vi "Test_PublishI32_PubBeforeSub_OK.vi"(8 "error in (no error)":errorcluster, 11 "TestMediator In":refnum<class "TestMediator.lvclass">) -> (0 "error out":errorcluster, 3 "TestMediator Out":refnum<class "TestMediator.lvclass">)   [LabVIEW 2015, in "TestMediator.lvclass"]
uses:
  TestMediator.lvclass
  Mediator/Mediator.lvclass
  Transport/QueueTransport/QueueTransport.lvclass/QueueTransport.ctl
  SubscriptionPolicy/BasicSubscription/BasicSubscription.lvclass/BasicSubscription.ctl
  IMediator/SubscriptionRequest/SubscriptionRequest.lvclass/SubscriptionRequest.ctl
  IMediator/IMediator Messages/Publish Msg/Publish Msg.lvclass/Publish Msg.ctl
  <vilib>/ActorFramework/Message Enqueuer/Message Enqueuer.lvclass/Message Enqueuer.ctl
  IMediator/IMediator Messages/Subscribe Msg/Subscribe Msg.lvclass/Subscribe Msg.ctl
  <vilib>/ActorFramework/Message Enqueuer/Enqueue.vi
  <vilib>/ActorFramework/Message Priority Queue/Priority Enqueue.vi
  <vilib>/Utility/error.llb/Error Cluster From Error Code.vi
  SubscriptionPolicy/BasicSubscription/BasicSubscription.lvclass
  IMediator/IMediator Messages/Publish Msg/Publish Msg.lvclass
  Transport/QueueTransport/QueueTransport.lvclass
  IMediator/SubscriptionRequest/SubscriptionRequest.lvclass
  IMediator/IMediator Messages/Subscribe Msg/Subscribe Msg.lvclass
  <vilib>/ActorFramework/Stop Msg/Stop Msg.lvclass
  <vilib>/addons/_JKI Toolkits/VI Tester/TestCase.llb/TestCase.lvclass
  <vilib>/ActorFramework/Actor/Actor.lvclass
  IMediator/ISubscriptionPolicy/ISubscriptionPolicy.lvclass
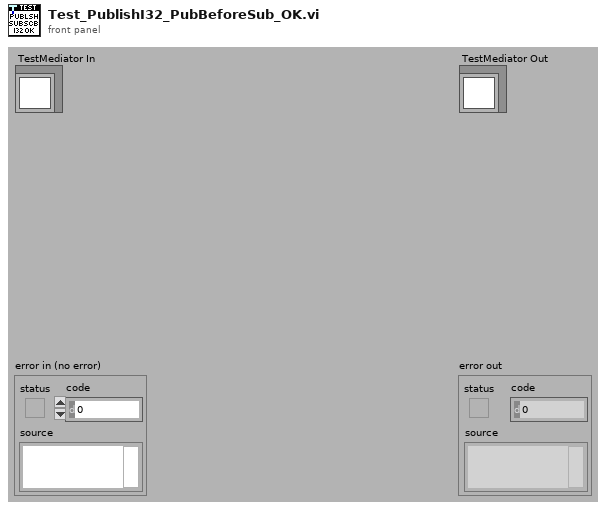
[diagram p1: front panel]
types:
  T1 = typedef "IMediator.lvlib/ISubscriptionPolicy.lvclass/ISubscriptionPolicy Reference.ctl" = refnum<data-value>
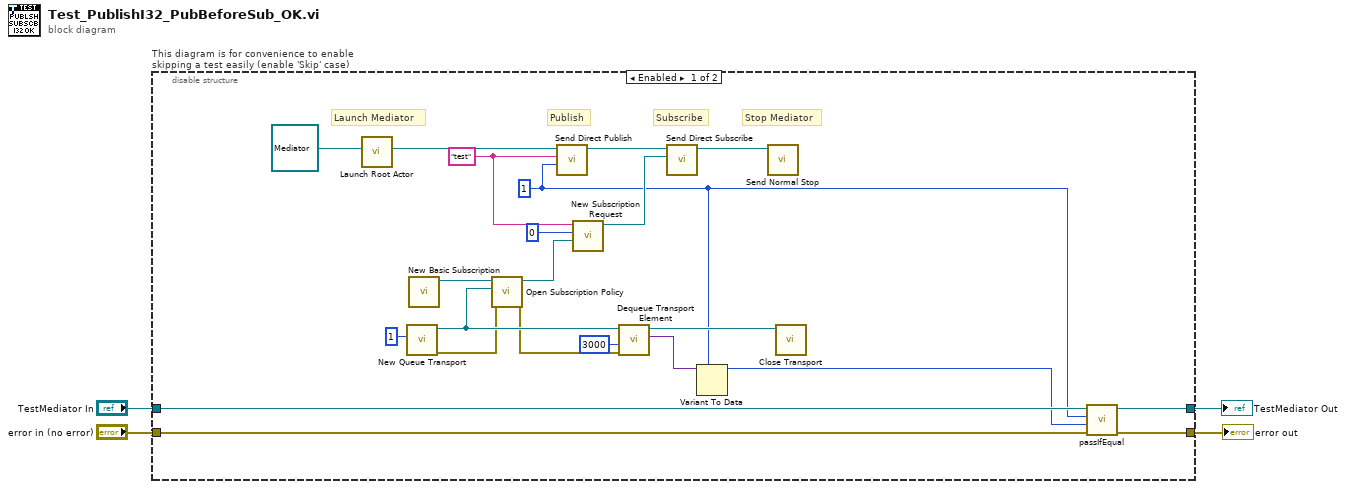
[diagram p0: block diagram]
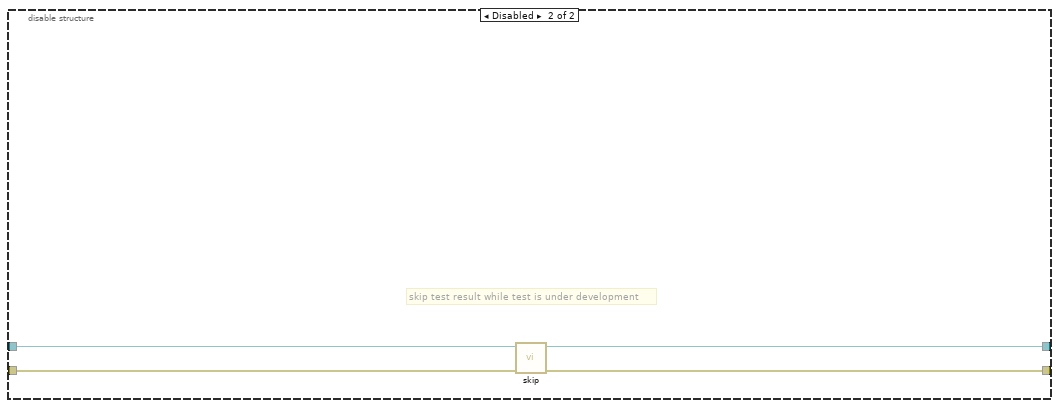
[diagram p2: hidden frame]
diagram:
  n1 = disable-structure "This diagram is for convenience to enable skipping a test easily (enable 'Skip' case)" shown="Enabled" {
    disable-tunnel: "TestMediator In" -> [w26 w30]
    disable-tunnel: [w25 w28] -> w1
    disable-tunnel: [w24 w29] -> w3
    disable-tunnel: "error in (no error)" -> [w23 w27]
    frame Enabled {
      w18 = "test" ("Datum Name")
      w8 = 1
      # "Launch Mediator"
      # "Stop Mediator"
      # "Subscribe"
      # "Publish"
      n2 = call <vilib>:"Launch Root Actor.vi"("Actor"=refnum<class "Mediator.lvclass"> refnum ("Mediator.lvlib:Mediator.lvclass")) -> ("Actor's Enqueuer"=w21:refnum<class "Message Enqueuer.lvclass">)  [unwired: 9 in, 1 out]
      n3 = call "New Queue Transport.vi"("Max Queue Size (-1)"=1) -> ("error out"=w13:errorcluster, "QueueTransport"=w15:refnum<class "QueueTransport.lvclass">)  [unwired: 9 in]
      n4 = call "New Basic Subscription.vi"() -> ("BasicSubscription Out"=w6:refnum<class "BasicSubscription.lvclass">)  [unwired: 11 in]
      n5 = call "Open Subscription Policy.vi"("error in (no error)"=w13, "Transport"=w15, "SubscriptionPolicy"=w6) -> ("error out"=w12:errorcluster, "Subscription Policy"=w5:T1)  [unwired: 7 in]
      n6 = call "Send Direct Publish.vi"("Data to Publish"=w8, "Datum Name"=w18, "Mediator Enqeuer"=w21) -> ("Mediator Enqueuer out"=w19:refnum<class "Message Enqueuer.lvclass">)  [unwired: 7 in, 1 out]
      n7 = call "New Subscription Request.vi"("Subscription Policy"=w5, "Type"=0, "Datum Name"=w18) -> ("SubscriptionRequest"=w20:refnum<class "SubscriptionRequest.lvclass">)  [unwired: 8 in]
      n8 = call "Dequeue Transport Element.vi"("error in (no error)"=w12, "Timeout In ms (-1)"=3000, "QueueTransport in"=w15) -> ("Data"=w9:variant, "QueueTransport out"=w10:refnum<class "QueueTransport.lvclass">)  [unwired: 5 in, 2 out]
      n9 = call "Send Direct Subscribe.vi"("Subscription Request"=w20, "Message Enqueuer"=w19) -> ("Message Enqueuer out"=w11:refnum<class "Message Enqueuer.lvclass">)  [unwired: 8 in, 1 out]
      n10 = Variant To Data(type=w8, Variant=w9) -> (data=w7:i32)  [unwired: 1 in, 1 out]
      n11 = call <vilib>:"Send Normal Stop.vi"("Message Enqueuer"=w11) -> ()  [unwired: 10 in, 1 out]
      n12 = call-dynamic "Close Transport.vi"("QueueTransport in"=w10) -> ()  [unwired: 10 in, 1 out]
      n13 = call-dynamic "passIfEqual.vi"("error in (no error)"=w23, "y"=w7, "x"=w8, "TestCase in"=w26) -> ("error out"=w24:errorcluster, "TestCase out"=w25:refnum<class "TestMediator.lvclass">)  [unwired: 6 in]
    }
    frame Disabled {
      # "skip test result while test is under development"
      n14 = call <vilib>:"skip.vi"("error in (no error)"=w27, "TestCase in"=w30) -> ("error out"=w29:errorcluster, "TestCase out"=w28:refnum<class "TestMediator.lvclass">)  [unwired: 8 in]
    }
  }
  "error out" <- w3
  "TestMediator Out" <- w1
